vi "Constellation Graph (SubVI).vi"(10 "Odd bits":dbl[](array[numeric]), 11 "Even bits":dbl[](array[numeric])) -> (3 "Constellation graph":cluster{"Y":dbl[], "Y":dbl[]}[](graph))   [LabVIEW 2026]
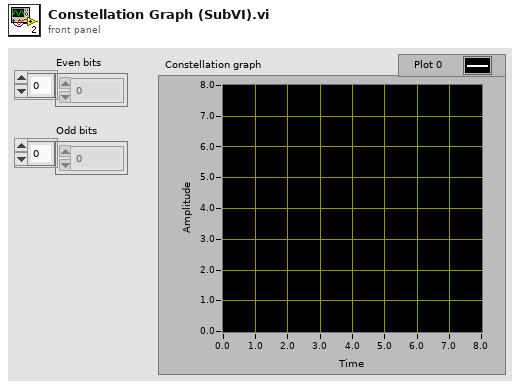
[diagram p1: front panel]
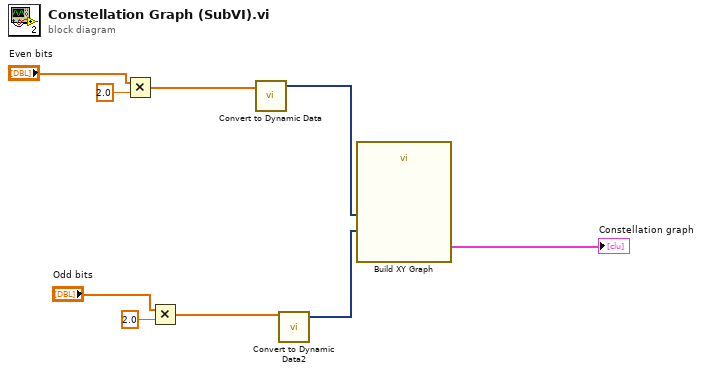
[diagram p0: block diagram]
diagram:
  n1 = Multiply(x="Even bits", y=2.0) -> (x*y=w3:dbl[])
  n2 = Multiply(x="Odd bits", y=2.0) -> (x*y=w4:dbl[])
  n3 = call "Convert to Dynamic Data"("Array"=w3) -> ("Dynamic Data Type"=w8:dynamicdata)  [unwired: 3 in]
  n4 = call "Convert to Dynamic Data2"("Array"=w4) -> ("Dynamic Data Type"=w9:dynamicdata)  [unwired: 3 in]
  n5 = call "Build XY Graph"("Y Input"=w9, "X Input"=w8) -> ("XY Graph"=→"Constellation graph":cluster{"X":dbl[], "Y":dbl[]}[])  [unwired: 8 in, 1 out]
